vi "explore-z-axis.vi"() -> ()   [LabVIEW 2015]
uses:
  <vilib>/rvi/Emulation/niFpgaGetClockAttributes.vi
  <vilib>/rvi/Emulation/niFpgaSctlEmulationGetInTimedLoop.vi
  <vilib>/rvi/Emulation/niFpgaEmulationReportErrorSimple.vi
  <vilib>/rvi/eio/common/nirviEmuTemplateMethod_errors.vi
  <vilib>/rvi/Emulation/niFpgaEmulationIsFPGAContextNoSignature.vi
  <vilib>/rvi/DataTransferAndStorage/Container/Common/niFpgaContainerGetUniqueNameForEmu.vi
  <vilib>/rvi/Memory/Memory_Emulation/niFpgaMemoryEmulationCacheClearOnFirstRun.vi
  <vilib>/rvi/Memory/Memory_Emulation/nirvimemoryEmulationManagerCache_MakeExclusive.vi
  <vilib>/rvi/Memory/Memory_Emulation/niFpgaMemoryEmulationValidateCache.vi
  <vilib>/rvi/Memory/Memory_Emulation/nirvimemoryEmulationManagerCache_InsertValue.vi
  <vilib>/Utility/error.llb/Clear Errors.vi
  <vilib>/rvi/Memory/Memory_Emulation/nirvimemoryEmulationManagerCache_ReleaseExclusive.vi
  <vilib>/rvi/Memory/Memory_Emulation/nirvimemoryEmulationManagerCache_GetValue.vi
  <vilib>/rvi/Memory/Memory_Emulation/nirvimemoryEmulationManagerCache_SetValue.vi
  <vilib>/rvi/Emulation/niFpgaProcessEmulError.vi
  <vilib>/rvi/Emulation/niFpgaCriticalErrorInLSC.vi
  <vilib>/eio/EIONode/EIONode.xnode
  <vilib>/rvi/DataTransferAndStorage/Container/XNode/niFpgaContainer.xnode
  <vilib>/rvi/DataTransferAndStorage/Register/Emulation/niFpgaRegisterEmulation.vi
  libimaging-cs.lvlib
panel:
  in  "case2 transition":i16=2
  out "Data":fxp<+/-,16,5>
  out "newcase":i16
  out "trigger":bool
  in  "unstable-excess":sgl=5.0
  out "AO2":sgl
  out "Mod2/AI2":fxp<+/-,24,5>
  in  "raise-constant":sgl
  in  "initial case":i16=2
  in  "Boolean 2":bool
  out "u-ramp":sgl
  in  "TOL":sgl=0.3 format="%#_13g"
  in  "u(0)":sgl format="%#_13g"
  in  "Force SP (v)":sgl
  in  "Ki":sgl
  in  "ramp-rate":sgl format="%#_13g"
  in  "Boolean":bool=TRUE
  in  "Cluster":cluster{"TsTicks":u32, "force setpoint":sgl}={"TsTicks"=1600, "force setpoint"=0.0}
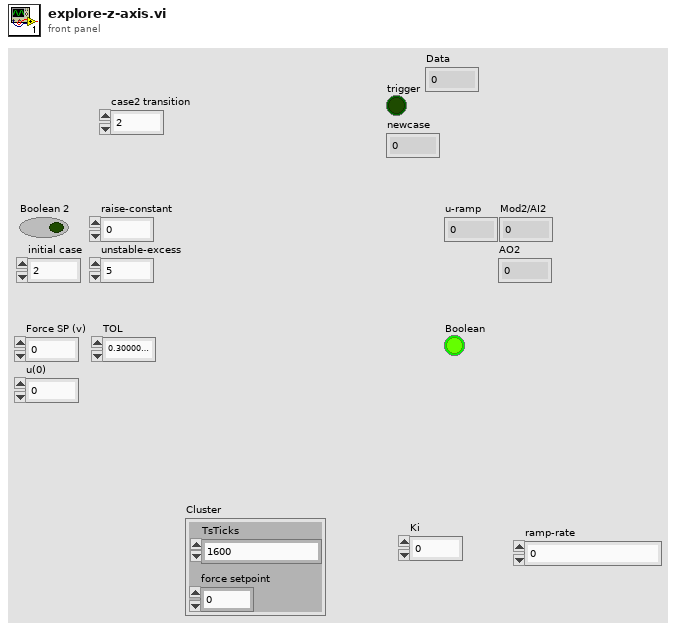
[diagram p1: front panel]
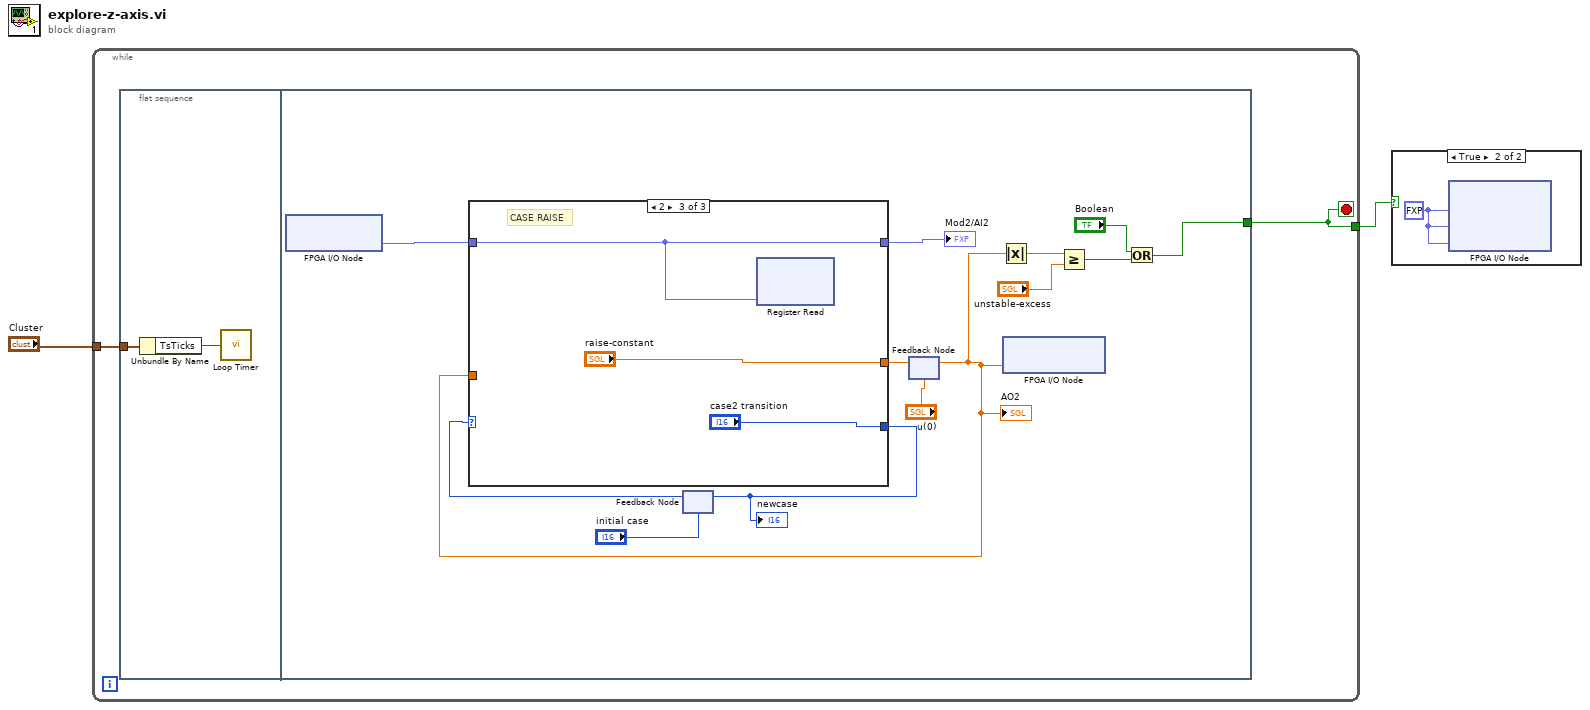
[diagram p0: block diagram]
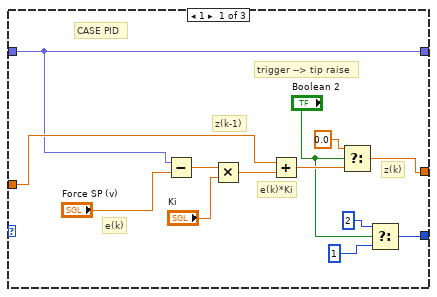
[diagram p3: hidden frame]
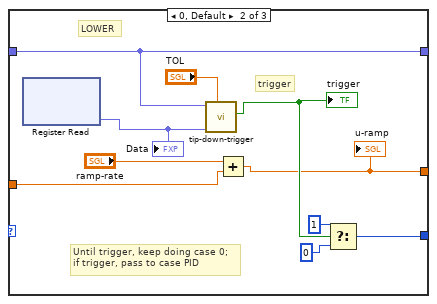
[diagram p4: hidden frame]
diagram:
  n1 = while {
    tunnel: [w4] -> w2
    tunnel: "Cluster" -> [w3]
    stop <- w4 stop-if-true
    n2 = flat-sequence {
      tunnel: w3 -> [w5]
      tunnel: [w12] -> w4
      frame #0 {
        n3 = Unbundle By Name(w5) -> ("TsTicks"=w6:u32)
        n4 = call "Loop Timer"("Count(Ticks)"=w6) -> ()  [unwired: 1 out]
      }
      frame #1 {
        n5 = xnode "FPGA I/O Node"() -> ("Mod2/AI2"=w18:fxp<+/-,24,5>)  [unwired: 1 in, 1 out]
        n6 = feedback #1("initial case") -> (w7:i16)
        n7 = feedback #2("u(0)") -> (w10:sgl)
        "AO2" <- w10
        n8 = case shown="2" w7 {
          tunnel: [w28 w33 "raise-constant"] -> w19
          tunnel: w10 -> [w22 w42 _]
          tunnel: w18 -> [w21 w37 w43]
          tunnel: [w21 w37 w43] -> w16
          tunnel: [w26 w39 "case2 transition"] -> w9
          frame 1 {
            # "trigger --> tip raise"
            # "z(k)"
            # "e(k)*Ki"
            # "z(k-1)"
            # "e(k)"
            # "CASE PID"
            n9 = Subtract(x=w21, y="Force SP (v)") -> (x-y=w31:sgl)
            n10 = Multiply(x=w31, y="Ki") -> (x*y=w30:sgl)
            n11 = Add(x=w22, y=w30) -> (x+y=w29:sgl)
            n12 = Select(t=sgl 0.0 ("f"), s="Boolean 2", f=w29) -> (s? t:f=w28:sgl)
            n13 = Select(t=i16 2, s="Boolean 2", f=i16 1) -> (s? t:f=w26:i16)
          }
          frame 0, Default {
            # "Until trigger, keep doing case 0;\nif trigger, pass to case PID"
            # "LOWER"
            # "trigger"
            n14 = xnode ("Register Read")() -> ("Data"=w34:fxp<+/-,16,5>)  [unwired: 1 in, 1 out]
            "Data" <- w34
            n15 = call "tip-down-trigger.vi"("TOL"="TOL", "Vo"=w34, "e(k)"=w37) -> ("trigger"=w35:bool)  [unwired: 8 in]
            "trigger" <- w35
            n16 = Add(x="ramp-rate", y=w42) -> (x+y=w33:sgl)
            "u-ramp" <- w33
            n17 = Select(t=i16 1, s=w35, f=i16 0) -> (s? t:f=w39:i16)
          }
          frame 2 {
            # "CASE RAISE"
            n18 = xnode ("Register Read")("Data"=w43) -> ()  [unwired: 1 in, 1 out]
          }
        }
        "Mod2/AI2" <- w16
        "newcase" <- w9
        n19 = feedback-in #1(w9) -> ()
        n20 = feedback-in #2(w19) -> ()
        n21 = Absolute Value(x=w10) -> (abs(x)=w11:sgl)
        n22 = xnode "FPGA I/O Node"("Mod1/AO2"=w10) -> ()  [unwired: 1 in, 1 out]
        n23 = Greater Or Equal?(x=w11, y="unstable-excess") -> (x >= y?=w14:bool)
        n24 = Or(x="Boolean", y=w14) -> (x .or. y?=w12:bool)
      }
    }
  }
  n25 = case shown="True" w2 {
    frame False {
    }
    frame True {
      w46 = fxp<+/-,20,5> 0.0 ("Mod1/AO0")
      n26 = xnode "FPGA I/O Node"("Mod1/AO0"=w46, "Mod1/AO1"=w46, "Mod1/AO2"=w46) -> ()  [unwired: 3 in, 3 out]
    }
  }
